vi "PhotonUtils_EstimateFieldToRobot.vi"(4 "CameraToRobot":T1={"TRANSLATION"={"X"=0.0, "Y"=0.0}, "ROTATION"={"VALUE"=0.0, "COS"=1.0, "SIN"=0.0}} {"ROTATION"."SIN" format="%13.4f"; "ROTATION"."COS" format="%13.4f"; "ROTATION"."VALUE" format="%13.4f"; "TRANSLATION"."Y" format="%14.3f"; "TRANSLATION"."X" format="%14.3f"}, 5 "cameraHeight_Meters":dbl, 6 "FieldToTarget":T4={"TRANSLATION"={"X"=0.0, "Y"=0.0}, "ROTATION"={"VALUE"=0.0, "COS"=1.0, "SIN"=0.0}} {"ROTATION"."SIN" format="%13.4f"; "ROTATION"."COS" format="%13.4f"; "ROTATION"."VALUE" format="%13.4f"; "TRANSLATION"."Y" format="%14.3f"; "TRANSLATION"."X" format="%14.3f"}, 7 "targetHeight_Meters":dbl, 8 "GyroAngle":T3={"VALUE"=0.0, "COS"=1.0, "SIN"=0.0} {"SIN" format="%13.4f"; "COS" format="%13.4f"; "VALUE" format="%13.4f"}, 9 "TargetYaw":T3={"VALUE"=0.0, "COS"=1.0, "SIN"=0.0} {"SIN" format="%13.4f"; "COS" format="%13.4f"; "VALUE" format="%13.4f"}, 10 "targetPitch_Radians":dbl, 11 "cameraPitch_Radians":dbl) -> (3 "EstimateFieldToRobot":T4={"TRANSLATION"={"X"=0.0, "Y"=0.0}, "ROTATION"={"VALUE"=0.0, "COS"=1.0, "SIN"=0.0}} {"ROTATION"."SIN" format="%13.4f"; "ROTATION"."COS" format="%13.4f"; "ROTATION"."VALUE" format="%13.4f"; "TRANSLATION"."Y" format="%14.3f"; "TRANSLATION"."X" format="%14.3f"})   [LabVIEW 2019, in "PhotonVisionLib.lvlib"]
doc: "Estimate the position of the robot in the field.\n\nInputs:\n - CameraHeightMeters The physical height of the camera off the floor in meters.\n - TargetHeightMeters The physical height of the target off the floor in meters. \n This should be the height of whatever is being targeted (i.e. if the targeting\n region is set to top, this should be the height of the top of the target).\n - CameraPitchRadians The pitch of the camera from the horizontal plane in \n radians. Positive values up.\n - TargetPitchRadians The pitch of the target in the camera's lens in radians. Positive\n values up.\n - TargetYaw The observed yaw of the target. Note that this *must* be \n CCW-positive, and Photon returns CW-positive.\n - GyroAngle The current robot gyro angle, likely from odometry.\n - FieldToTarget A Pose2d representing the target position in the field coordinate \n system.\n - CameraToRobot The position of the robot relative to the camera. If the camera \n was mounted 3 inches behind the \"origin\" (usually physical center) of the\n robot, this would be Transform2d (3 inches, 0 inches, 0 degrees).\n\nOutputs\n - EstimateFieldToRobot -- The position of the robot in the field."
uses:
  PhotonVisionLib.lvlib
  <vilib>/Rock Robotics/WPI/ThirdParty/JAS_Junk/TrajLib/POSE2D.ctl
  <vilib>/Rock Robotics/WPI/ThirdParty/JAS_Junk/TrajLib/TRANSLATION2D.ctl
  <vilib>/Rock Robotics/WPI/ThirdParty/JAS_Junk/TrajLib/ROTATION2D.ctl
  <vilib>/Rock Robotics/WPI/ThirdParty/JAS_Junk/TrajLib/TRANSFORM2D.ctl
  <vilib>/Rock Robotics/WPI/ThirdParty/JAS_Junk/TrajLib/Trajectory_Library.lvlib
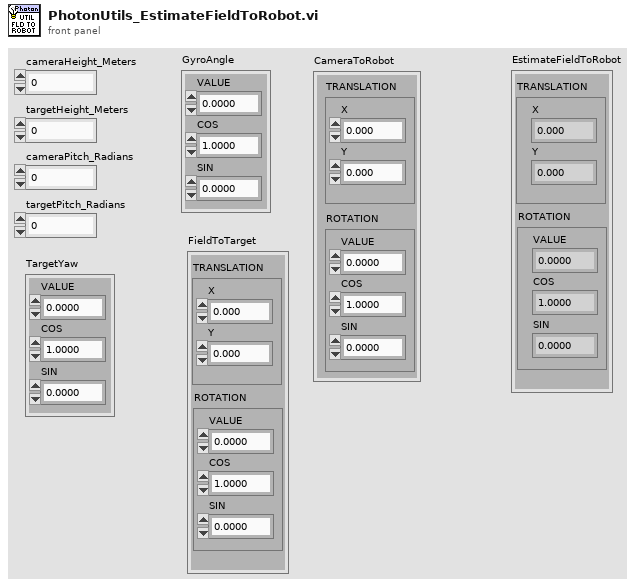
[diagram p1: front panel]
types:
  T1 = typedef "Trajectory_Library.lvlib/TRANSFORM2D.ctl" = cluster{"TRANSLATION":T2, "ROTATION":T3}
  T2 = typedef "Trajectory_Library.lvlib/TRANSLATION2D.ctl" = cluster{"X":dbl, "Y":dbl}
  T3 = typedef "Trajectory_Library.lvlib/ROTATION2D.ctl" = cluster{"VALUE":dbl, "COS":dbl, "SIN":dbl}
  T4 = typedef "Trajectory_Library.lvlib/POSE2D.ctl" = cluster{"TRANSLATION":T2, "ROTATION":T3}
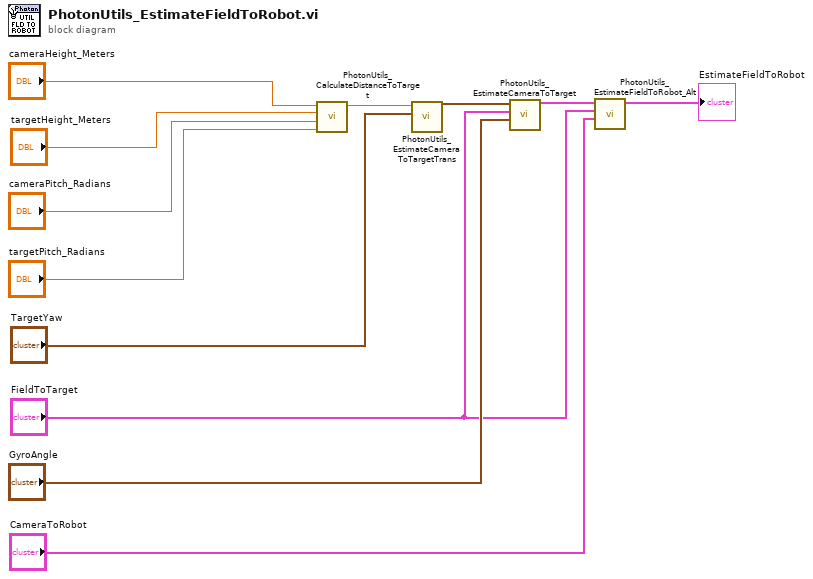
[diagram p0: block diagram]
diagram:
  n1 = call "PhotonUtils_CalculateDistanceToTarget.vi"("TargetPitch_Radians"="targetPitch_Radians", "CameraPitch_Radians"="cameraPitch_Radians", "TargetHeight_Meters"="targetHeight_Meters", "CameraHeight_Meters"="cameraHeight_Meters") -> ("DistanceToTarget_Meters"=w8:dbl)  [unwired: 7 in]
  n2 = call "PhotonUtils_EstimateCameraToTargetTrans.vi"("Yaw"="TargetYaw", "TargetDistance_Meters"=w8) -> ("CameraToTarget"=w6:T2)  [unwired: 9 in]
  n3 = call "PhotonUtils_EstimateCameraToTarget.vi"("GyroAngle"="GyroAngle", "FieldToTarget"="FieldToTarget", "CameraToTargetTranslation"=w6) -> ("estimateCameraToTarget"=w4:T1)  [unwired: 8 in]
  n4 = call "PhotonUtils_EstimateFieldToRobot_Alt.vi"("CameraToRobot"="CameraToRobot", "FieldToTarget"="FieldToTarget", "CameraToTarget,"=w4) -> ("EstimateFieldToRobot"=→"EstimateFieldToRobot":T4)  [unwired: 8 in]
